vi "nipkg-createFolders.vi"(8 "error in (no error)":errorcluster, 11 "New package source directory":path) -> (0 "error out":errorcluster, 3 "Package source directory out":path)   [LabVIEW 2014, in "nipkg-build-system.lvlib"]
uses:
  nipkg-build-system.lvlib
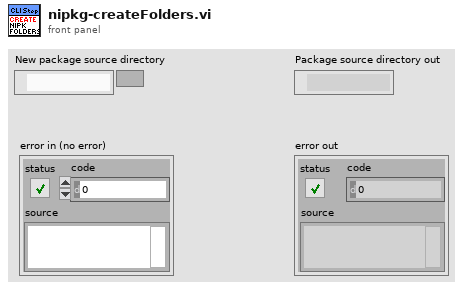
[diagram p1: front panel]
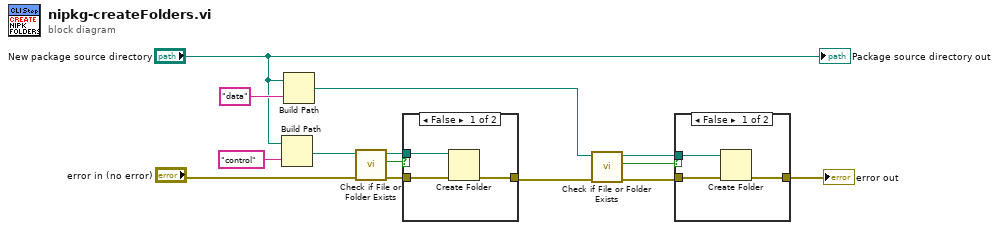
[diagram p0: block diagram]
diagram:
  n1 = Build Path(base path="New package source directory", name or relative path="control") -> (appended path=w10:path)
  n2 = Build Path(base path="New package source directory", name or relative path="data") -> (appended path=w5:path)
  n3 = call <vilib>:"Check if File or Folder Exists.vi"("error in (no error)"="error in (no error)", "path"=w10) -> ("error out"=w8:errorcluster, "file or folder exists?"=w9:bool, "dup path"=w2:path)  [unwired: 7 in]
  n4 = case shown="False" w9 {
    tunnel: w8 -> [w17 w18]
    tunnel: [w16 w18] -> w6
    tunnel: w2 -> [w15 _]
    frame False {
      n5 = Create Folder(path (use dialog)=w15, error in=w17) -> (error out=w16:errorcluster)  [unwired: 1 in, 2 out]
    }
    frame True {
    }
  }
  n6 = call <vilib>:"Check if File or Folder Exists.vi"("error in (no error)"=w6, "path"=w5) -> ("error out"=w4:errorcluster, "file or folder exists?"=w3:bool, "dup path"=w1:path)  [unwired: 7 in]
  n7 = case shown="False" w3 {
    tunnel: w4 -> [w21 w22]
    tunnel: [w20 w22] -> w7
    tunnel: w1 -> [w19 _]
    frame False {
      n8 = Create Folder(path (use dialog)=w19, error in=w21) -> (error out=w20:errorcluster)  [unwired: 1 in, 2 out]
    }
    frame True {
    }
  }
  "error out" <- w7
  "Package source directory out" <- "New package source directory"
